vi "jsonInsertDbl.vi"(8 "error in (no error)":errorcluster, 9 "value":dbl, 10 "path":string, 11 "d in":i64) -> (0 "error out":errorcluster, 3 "d out":i64)   [LabVIEW 2015, in "rapidjson wrapper.lvlib"]
uses:
  rapidjson wrapper.lvlib
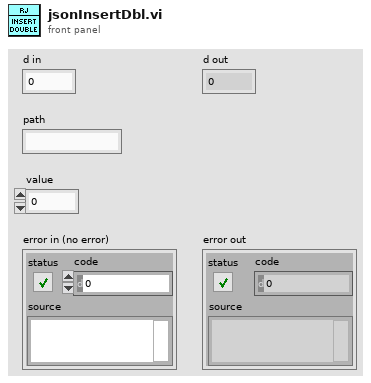
[diagram p1: front panel]
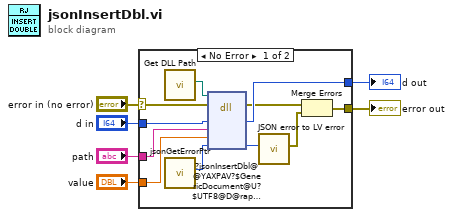
[diagram p0: block diagram]
diagram:
  n1 = case shown="No Error" "error in (no error)" {
    selector: "error in (no error)" -> [w10 w19]
    tunnel: [w7 w19] -> w6
    tunnel: "value" -> [w14 _]
    tunnel: "d in" -> [w13 w18]
    tunnel: "path" -> [w12 _]
    tunnel: [w11 w18] -> w1
    frame No Error {
      n2 = call "Get DLL Path.vi"() -> ("Path"=w17:path)  [unwired: 11 in]
      n3 = call "jsonGetErrorPtr.vi"() -> ("return type"=w15:i64)  [unwired: 10 in, 1 out]
      n4 = dll-call lib="C:/Users/tblair/Documents/Git Projects/LVrapidjson core/lvrjs/Debug/lvrjs.dll" fn="?jsonInsertDbl@@YAXPAV?$GenericDocument@U?$UTF8@D@rapidjson@@V?$MemoryPoolAllocator@VCrtAllocator@rapidjson@@@2@VCrtAllocator@2@@rapidjson@@PADN0@Z"(path in=w17, error in=w10, "d"=w13, "path"=w12, "value"=w14, "jsonError"=w15) -> (error out=w9:errorcluster, "d"=w11:i64, "jsonError"=w16:i64)  [unwired: 4 in, 1 out]
      n5 = call "JSON error to LV error.vi"("jsonError"=w16) -> ("error out"=w8:errorcluster)  [unwired: 10 in]
      n6 = Merge Errors(w9, w8) -> (w7:errorcluster)
    }
    frame Error {
    }
  }
  "error out" <- w6
  "d out" <- w1
